vi "AG Main.vi"() -> ()   [LabVIEW 2012]
uses:
  <userlib>/H_Utilities/myDAQ_State.ctl
  <vilib>/Platform/browser.llb/Open URL in Default Browser (string).vi
  <userlib>/H_Utilities/myDAQmx/myDAQmx Create Channel/Create myDAQ AI.vi
  <userlib>/H_Utilities/myDAQmx/myDAQmx Create Channel/Create myDAQ DO.vi
  <userlib>/H_Utilities/myDAQmx/myDAQmx Read/myDAQmx Read Analog Value.vi
  <userlib>/H_Utilities/myDAQmx/myDAQmxWrite/myDAQmx Write Digital - 1 Chan.vi
panel:
  in  "LabVIEW":bool
  in  "Report Issue":bool
  out "Error Out":errorcluster
  out "Event Loop":i32
  out "DAQ Loop":i32
  out "Active State":T1
  in  "AG Tabs":enum32{"Tab 1", "Tab 2", "Tab 3"}(tab)
  in  "Configure":bool
  in  "Measure":bool
  in  "AG Page Buttons":enum32{"Page 1", "Page 2", "Page 3", "Page 4"}(radio)
  in  "AG Pages":enum32{"Page 1", "Page 2", "Page 3", "Page 4"}(tab)
  in  "Get Started":bool
  out "Connected":bool
  in  "Tab Buttons":enum32{"Tab1", "Tab2", "Tab3"}(radio)
  # "Lab Title"
  # "1. Connect myDAQ to this computer.\n\n2. Connect the circuit as shown here."
  # "1. Calibrate your device"
  # "Measure"
  # "Getting Started Instructions"
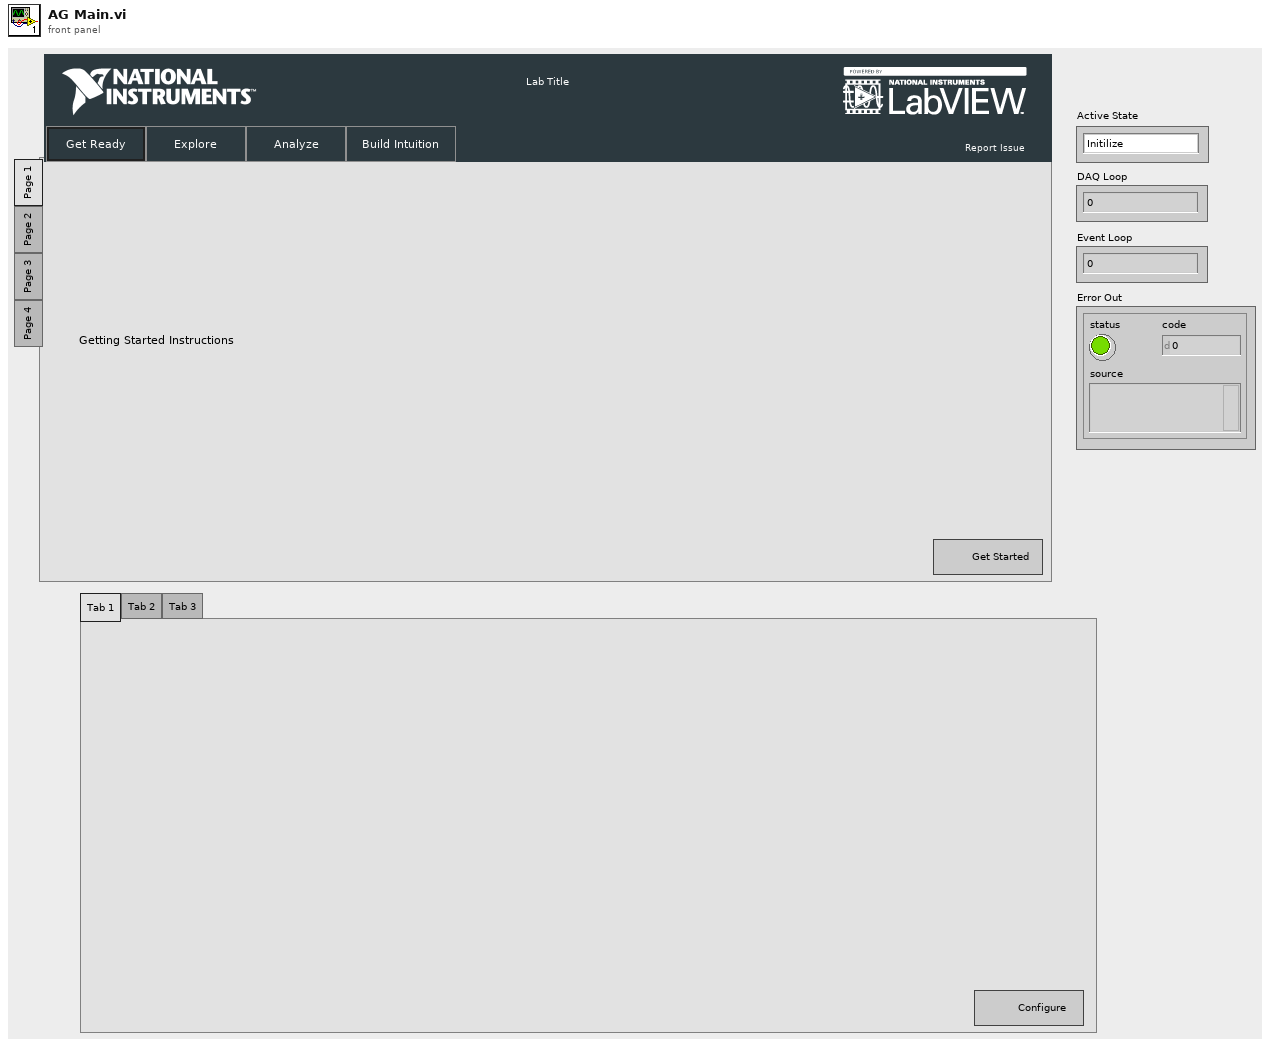
[diagram p1: front panel]
types:
  T1 = typedef "myDAQ_State.ctl" = enum16{"Initilize", "Connect", "Calibrate", "Communicate", "Wait", "Disconnect", "Error", "Close"}
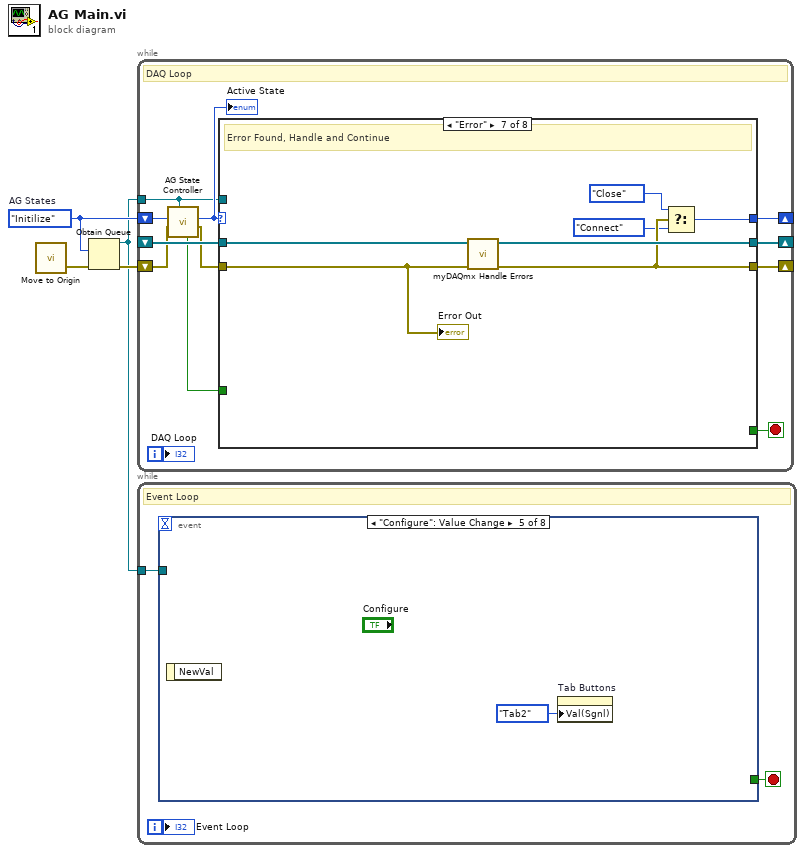
[diagram p0: block diagram]
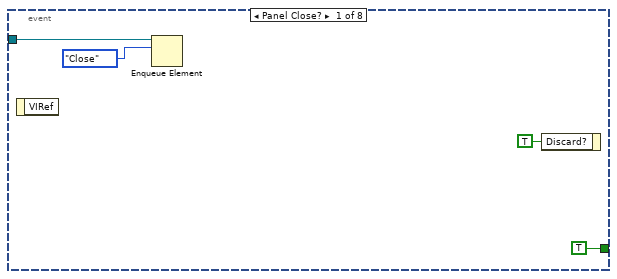
[diagram p2: hidden frame]
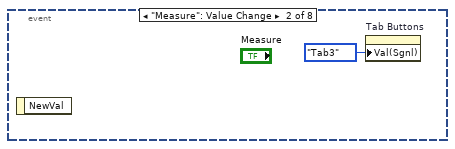
[diagram p3: hidden frame]
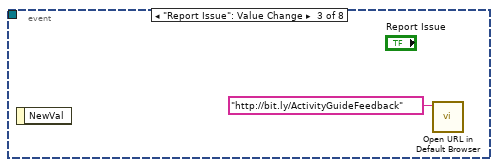
[diagram p4: hidden frame]
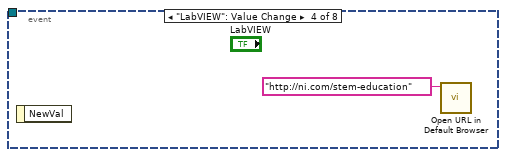
[diagram p5: hidden frame]
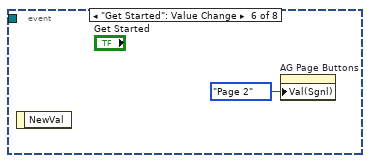
[diagram p6: hidden frame]
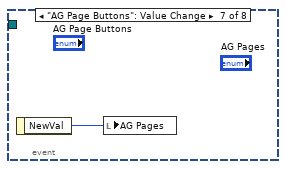
[diagram p7: hidden frame]
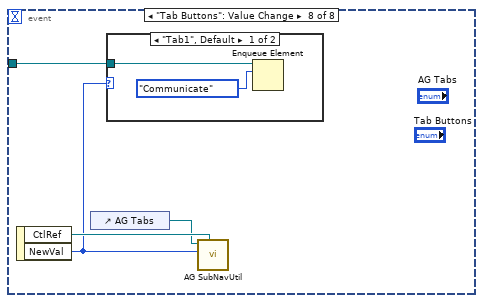
[diagram p8: hidden frame]
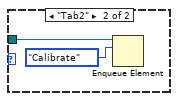
[diagram p9: hidden frame]
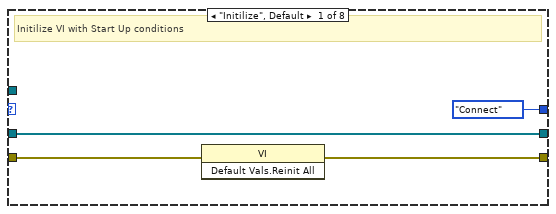
[diagram p10: hidden frame]
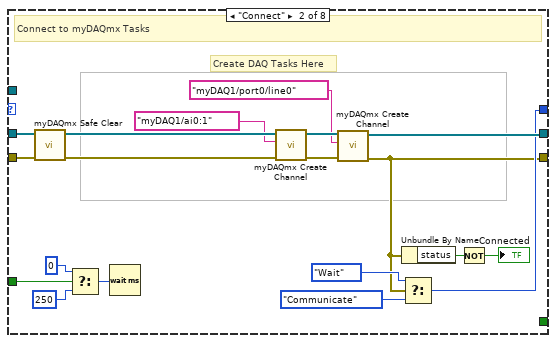
[diagram p11: hidden frame]
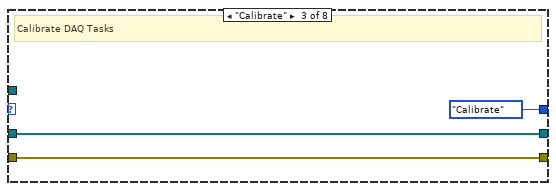
[diagram p12: hidden frame]
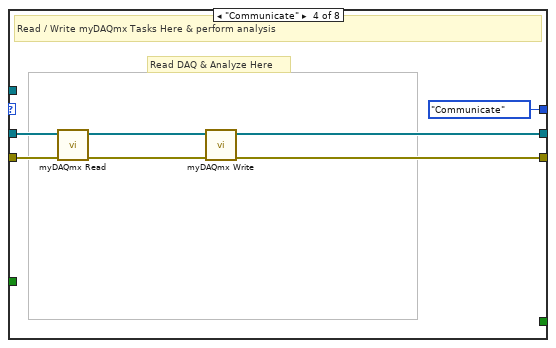
[diagram p13: hidden frame]
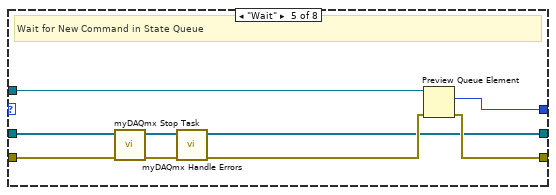
[diagram p14: hidden frame]
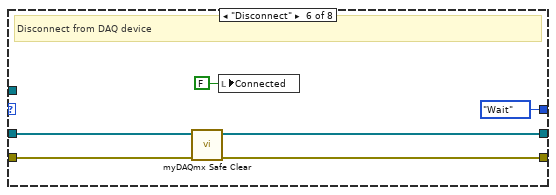
[diagram p15: hidden frame]
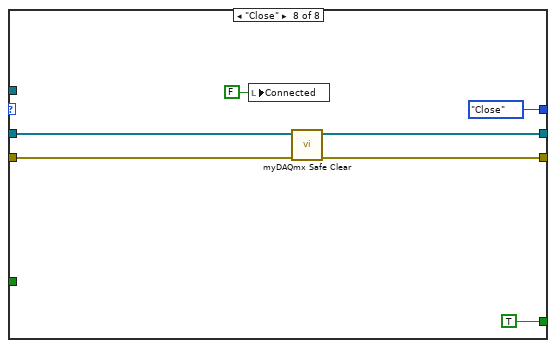
[diagram p16: hidden frame]
diagram:
  w4 = myDAQ_State."Initilize"  # AG States
  n1 = call "Move to Origin.vi"() -> ("Error Out"=w1:errorcluster)  [unwired: 3 in]
  n2 = Obtain Queue(element data type=w4, error in (no error)=w1) -> (queue out=w2:refnum<queue>, error out=w3:errorcluster)  [unwired: 3 in, 1 out]
  n3 = while {
    shift-right: [w16] -> _
    shift-left: _ -> [w14]
    shift-right: [w9] -> _
    shift-left: w4 -> [w13]
    tunnel: w2 -> [w6]
    shift-right: [w15] -> _
    shift-left: w3 -> [w12]
    i -> [w5]
    stop <- w7 stop-if-true
    # "DAQ Loop"
    n4 = call "AG State Controller.vi"("queue Ref"=w6, "Error In"=w12, "Default State"=w13) -> ("Error Out"=w11:errorcluster, "State Out"=w8:T1, "New State"=w10:bool)  [unwired: 6 in]
    "Active State" <- w8
    n5 = case shown="\"Error\"" w8 {
      tunnel: [w20 w32 w42 w43 w50 w62 w69 w77] -> w16
      tunnel: [w17 w24 w41 w44 w57 w61 w68 w76] -> w15
      tunnel: w14 -> [w20 w38 w42 w49 w54 w64 w71 w75]
      tunnel: w11 -> [w18 w37 w41 w48 w53 w63 w70 w74]
      tunnel: w10 -> [_ w31 _ _ _ _ _ _]
      tunnel: [myDAQ_State."Connect" ("AG States") w25 myDAQ_State."Calibrate" ("AG States") myDAQ_State."Communicate" ("AG States") w51 myDAQ_State."Wait" ("AG States") w65 myDAQ_State."Close" ("AG States")] -> w9
      tunnel: [_ _ _ _ _ _ _ TRUE] -> w7
      tunnel: w6 -> [_ _ _ _ w58 _ _ _]
      frame "Initilize", Default {
        # "Initilize VI with Start Up conditions"
        n6 = invoke class="VI" method="Default Vals.Reinit All"(error in=w18) -> (error out=w17:errorcluster)  [unwired: 2 in, 2 out]
      }
      frame "Connect" {
        # "Create DAQ Tasks Here"
        # "Connect to myDAQmx Tasks"
        n7 = call <userlib>:"myDAQmx Safe Clear.vi"("error in (no error)"=w37, "task array in"=w38) -> ("error out"=w36:errorcluster, "task array out"=w39:refnum<k21>[])  [unwired: 8 in]
        n8 = Select(t=u32 0 ("milliseconds to wait"), s=w31, f=u32 250 ("milliseconds to wait")) -> (s? t:f=w28:u32)
        n9 = Wait (ms)(milliseconds to wait=w28) -> ()  [unwired: 1 out]
        n10 = call-poly <userlib>:"myDAQmx Create Channel.vi"("error in (no error)"=w36, "physical channels (ai0:1)"=tag "myDAQ1/ai0:1", "task array in (none)"=w39) -> ("error out"=w34:errorcluster, "task array out"=w33:refnum<k21>[])  [unwired: 7 in]
        n11 = call-poly <userlib>:"myDAQmx Create Channel.vi"("error in (no error)"=w34, "lines (port0/line0)"=tag "myDAQ1/port0/line0", "task array in (none)"=w33) -> ("error out"=w24:errorcluster, "task array out"=w32:refnum<k21>[])  [unwired: 7 in]
        n12 = Unbundle By Name(w24) -> ("status"=w23:bool)
        n13 = Select(t=myDAQ_State."Wait" ("AG States"), s=w24, f=myDAQ_State."Communicate" ("AG States")) -> (s? t:f=w25:T1)
        n14 = Not(x=w23) -> (.not. x?=→"Connected":bool)
      }
      frame "Calibrate" {
        # "Calibrate DAQ Tasks"
      }
      frame "Communicate" {
        # "Read DAQ & Analyze Here"
        # "Read / Write myDAQmx Tasks Here & perform analysis"
        n15 = call-poly <userlib>:"myDAQmx Read.vi"("error in (no error)"=w48, "task array in"=w49) -> ("error out"=w45:errorcluster, "task array out"=w46:refnum<k21>[])  [unwired: 6 in, 2 out]
        n16 = call-poly <userlib>:"myDAQmx Write.vi"("error in (no error)"=w45, "task array in"=w46) -> ("error out"=w44:errorcluster, "task array out"=w43:refnum<k21>[])  [unwired: 8 in]
      }
      frame "Wait" {
        # "Wait for New Command in State Queue"
        n17 = call <userlib>:"myDAQmx Stop Task.vi"("error In"=w53, "task array in"=w54) -> ("Error Out"=w55:errorcluster, "task array out"=w56:refnum<k21>[])  [unwired: 8 in]
        n18 = call <userlib>:"myDAQmx Handle Errors.vi"("Error In"=w55, "Task Array In"=w56) -> ("Error Out"=w52:errorcluster, "Task Array Out"=w50:refnum<k21>[])  [unwired: 6 in, 2 out]
        n19 = Preview Queue Element(queue=w58, error in (no error)=w52) -> (element=w51:T1, error out=w57:errorcluster)  [unwired: 1 in, 2 out]
      }
      frame "Disconnect" {
        # "Disconnect from DAQ device"
        n20 = call <userlib>:"myDAQmx Safe Clear.vi"("error in (no error)"=w63, "task array in"=w64) -> ("error out"=w61:errorcluster, "task array out"=w62:refnum<k21>[])  [unwired: 8 in]
        n21 = local write "Connected"(FALSE ("Connected")) -> ()
      }
      frame "Error" {
        # "Error Found, Handle and Continue"
        n22 = call <userlib>:"myDAQmx Handle Errors.vi"("Error In"=w70, "Task Array In"=w71) -> ("Error Out"=w68:errorcluster, "Task Array Out"=w69:refnum<k21>[])  [unwired: 6 in, 2 out]
        n23 = Select(t=myDAQ_State."Close" ("AG States"), s=w68, f=myDAQ_State."Connect" ("AG States")) -> (s? t:f=w65:T1)
        "Error Out" <- w70
      }
      frame "Close" {
        n24 = local write "Connected"(FALSE ("Connected")) -> ()
        n25 = call <userlib>:"myDAQmx Safe Clear.vi"("error in (no error)"=w74, "task array in"=w75) -> ("error out"=w76:errorcluster, "task array out"=w77:refnum<k21>[])  [unwired: 8 in]
      }
    }
    "DAQ Loop" <- w5
  }
  n26 = while {
    tunnel: w2 -> [w81]
    i -> [w79]
    stop <- w80 stop-if-true
    # "Event Loop"
    n27 = event shown="[4] \"Configure\": Value Change" {
      selector: _ -> [_ _ _ _ _ _ _ _]
      dyn-events: _ -> [_ _ _ _ _ _ _ _]
      timeout: _ -> [_ _ _ _ _ _ _ _]
      tunnel: w81 -> [w85 _ _ _ _ _ _ w92]
      tunnel: [TRUE _ _ _ _ _ _ _] -> w80
      event Panel Close? {
        n28 = event-data() -> ()  [unwired: 1 in, 1 out]
        n29 = Enqueue Element(queue=w85, element=myDAQ_State."Close") -> ()  [unwired: 2 in, 3 out]
        n30 = event-data("Discard?"=TRUE) -> ()  [unwired: 1 in, 1 out]
      }
      event "Measure": Value Change {
        n31 = event-data() -> ()  [unwired: 1 in, 1 out]
        n32 = property on="Tab Buttons" class="RadioBtnsControl (strict)"("Val(Sgnl)"=enum32{"Tab1", "Tab2", "Tab3"}."Tab3" ("Value (Signaling)")) -> ()  [unwired: 2 in, 2 out]
      }
      event "Report Issue": Value Change {
        n33 = event-data() -> ()  [unwired: 1 in, 1 out]
        n34 = call-poly <vilib>:"Open URL in Default Browser.vi"("URL"="http://bit.ly/ActivityGuideFeedback") -> ()  [unwired: 5 in, 2 out]
      }
      event "LabVIEW": Value Change {
        n35 = event-data() -> ()  [unwired: 1 in, 1 out]
        n36 = call-poly <vilib>:"Open URL in Default Browser.vi"("URL"="http://ni.com/stem-education") -> ()  [unwired: 5 in, 2 out]
      }
      event "Configure": Value Change {
        n37 = event-data() -> ()  [unwired: 1 in, 1 out]
        n38 = property on="Tab Buttons" class="RadioBtnsControl (strict)"("Val(Sgnl)"=enum32{"Tab1", "Tab2", "Tab3"}."Tab2" ("Value (Signaling)")) -> ()  [unwired: 2 in, 2 out]
      }
      event "Get Started": Value Change {
        n39 = event-data() -> ()  [unwired: 1 in, 1 out]
        n40 = property on="AG Page Buttons" class="RadioBtnsControl (strict)"("Val(Sgnl)"=enum32{"Page 1", "Page 2", "Page 3", "Page 4"}."Page 2" ("Value (Signaling)")) -> ()  [unwired: 2 in, 2 out]
      }
      event "AG Page Buttons": Value Change {
        n41 = event-data() -> ("NewVal"=w91:enum32{"Page 1", "Page 2", "Page 3", "Page 4"})  [unwired: 1 in]
        n42 = local write "AG Pages"(w91) -> ()
      }
      event "Tab Buttons": Value Change {
        n43 = event-data() -> ("CtlRef"=w95:refnum<vi>, "NewVal"=w93:enum32{"Tab1", "Tab2", "Tab3"})  [unwired: 1 in]
        n44 = control-ref of="AG Tabs"() -> (w94:refnum<vi>)
        n45 = case shown="\"Tab1\", Default" w93 {
          tunnel: w92 -> [w96 w98]
          frame "Tab1", Default {
            n46 = Enqueue Element(queue=w96, element=myDAQ_State."Communicate") -> ()  [unwired: 2 in, 3 out]
          }
          frame "Tab2" {
            n47 = Enqueue Element(queue=w98, element=myDAQ_State."Calibrate") -> ()  [unwired: 2 in, 3 out]
          }
        }
        n48 = call "AG SubNavUtil.vi"("Progress Ref"=w95, "NewVal"=w93, "Tab Ref"=w94) -> ()  [unwired: 8 in, 1 out]
      }
    }
    "Event Loop" <- w79
  }
